vi "DAQ Configuration.vi"(8 "error in (no error)":errorcluster caption="错误输入（无错误）", 11 "parameter input":T1) -> (0 "error out":errorcluster caption="错误输出", 3 "parameter output":T1)   [LabVIEW 2015, in "DAQ.lvlib"]
doc: "该模板用于创建子VI。"
uses:
  DAQ.lvlib
  DAQ Configuration.ctl
  Utility VIs/Utility VIs.lvlib
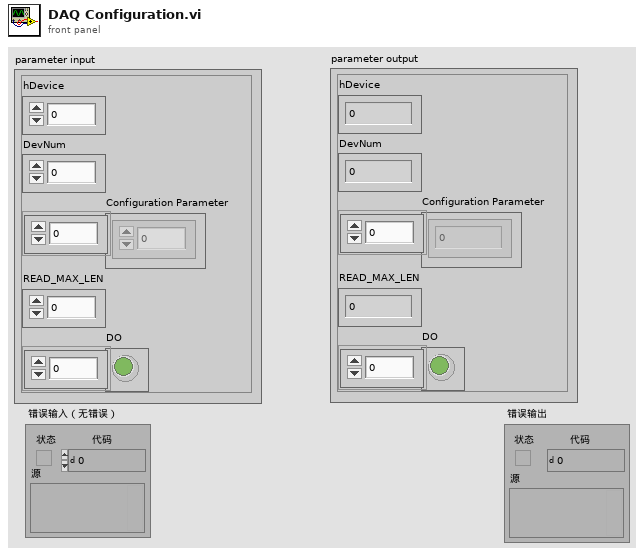
[diagram p1: front panel]
types:
  T1 = typedef "DAQ.lvlib/DAQ Configuration.ctl" = cluster{"hDevice":i32, "DevNum":u8, "Configuration Parameter":i32[], "READ_MAX_LEN":i32, "DO":bool[]}
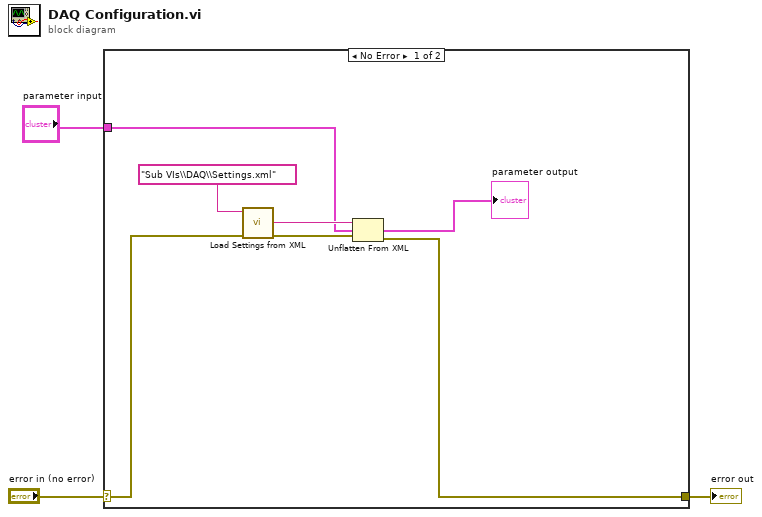
[diagram p0: block diagram]
diagram:
  n1 = case shown="No Error" "error in (no error)" {
    selector: "error in (no error)" -> [w6 w11]
    tunnel: [w5 w11] -> w2
    tunnel: "parameter input" -> [w8 _]
    frame No Error {
      n2 = call "Load Settings from XML.vi"("error in (no error)"=w6, "名称或相对路径"="Sub VIs\\DAQ\\Settings.xml") -> ("error out"=w7:errorcluster, "XML Elements"=w9:string)  [unwired: 8 in]
      n3 = Unflatten From XML(xml string=w9, type=w8, error in (no error)=w7) -> (value=→"parameter output":T1, error out=w5:errorcluster)
    }
    frame Error {
    }
  }
  "error out" <- w2
